vi "Parse Bucket Notification.vi"(11 "Notification Parameters":T1) -> (3 "PUT Data":string)   [LabVIEW 2015, in "NI_AWS_S3.lvlib"]
uses:
  NI_AWS_S3.lvlib
  Notification Configuration.ctl
  Topic Configuration.ctl
  Event.ctl
  Core/HTTP Request/Name Value Pair.ctl
  Cloud Function Configuration.ctl
  Queue Configuration.ctl
  Core/HTTP Request/HTTP Request.lvclass
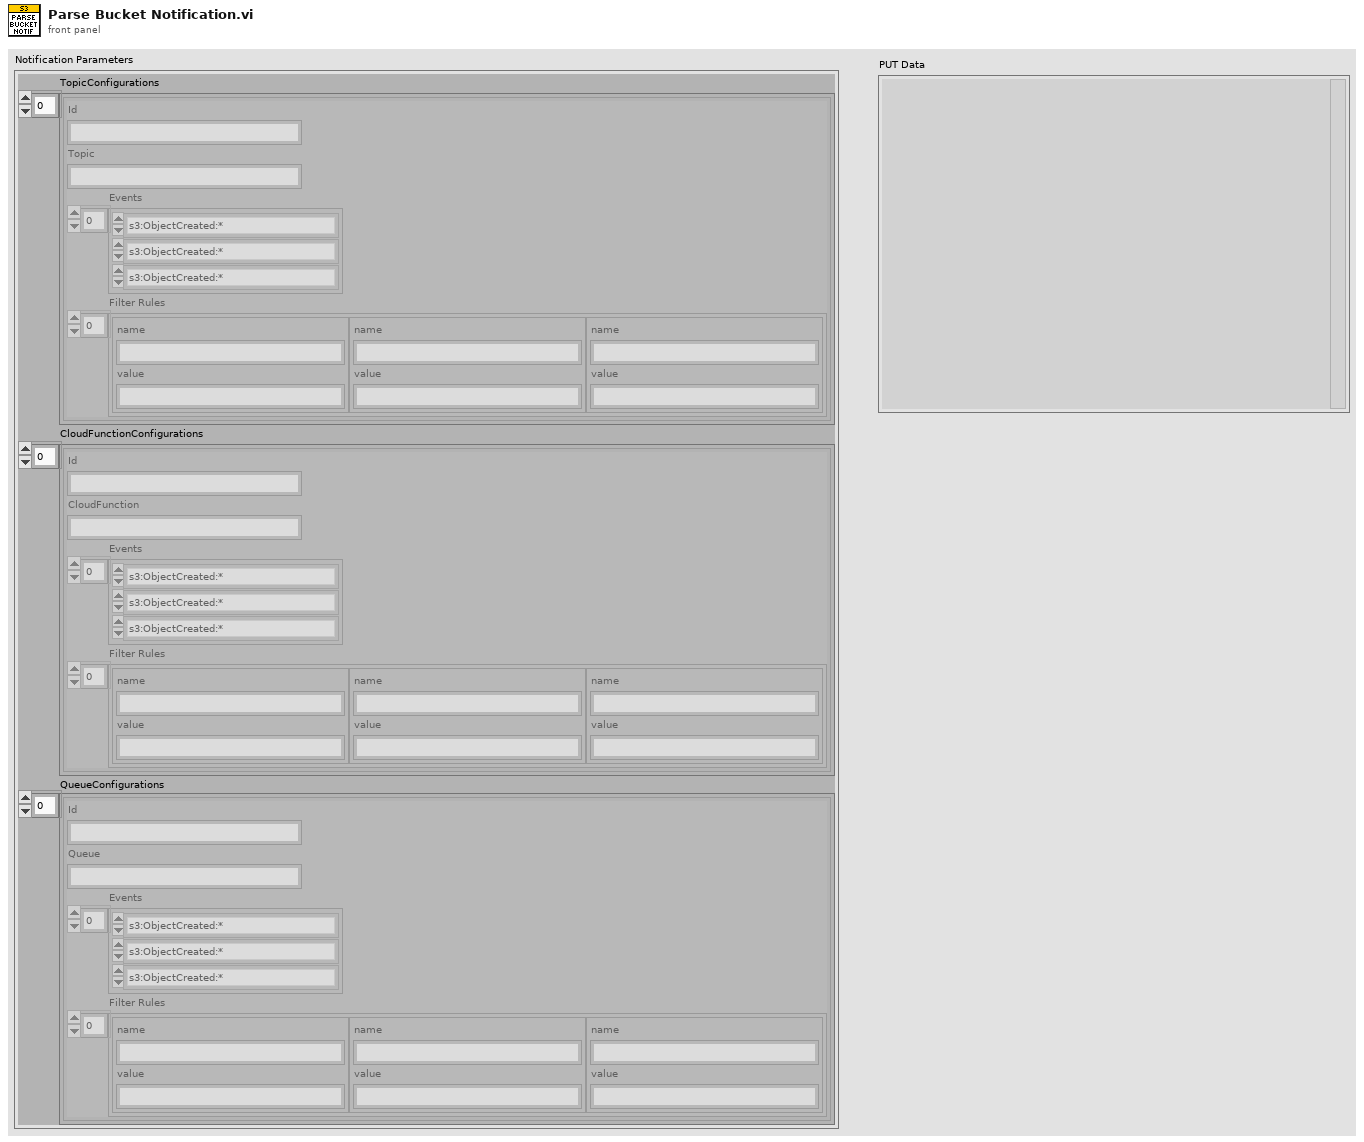
[diagram p1: front panel]
types:
  T1 = typedef "NI_AWS_S3.lvlib/Notification Configuration.ctl" = cluster{"TopicConfigurations":T2[], "CloudFunctionConfigurations":T5[], "QueueConfigurations":T6[]}
  T2 = typedef "NI_AWS_S3.lvlib/Topic Configuration.ctl" = cluster{"Id":string, "Topic":string, "Events":T3[], "Filter Rules":T4[]}
  T3 = typedef "NI_AWS_S3.lvlib/Event.ctl" = enum16{"s3:ObjectCreated:*", "s3:ObjectCreated:Put", "s3:ObjectCreated:Post", "s3:ObjectCreated:Copy", "s3:ObjectCreated:CompleteMultipartUpload", "s3:ObjectRemoved:*", "s3:ObjectRemoved:Delete", "s3:ObjectRemoved:DeleteMarkerCreated", "s3:ReducedRedundancyLostObject"}
  T4 = typedef "NI_AWS_Core.lvlib/HTTP Request.lvclass/Name Value Pair.ctl" = cluster{"name":string, "value":string}
  T5 = typedef "NI_AWS_S3.lvlib/Cloud Function Configuration.ctl" = cluster{"Id":string, "CloudFunction":string, "Events":T3[], "Filter Rules":T4[]}
  T6 = typedef "NI_AWS_S3.lvlib/Queue Configuration.ctl" = cluster{"Id":string, "Queue":string, "Events":T3[], "Filter Rules":T4[]}
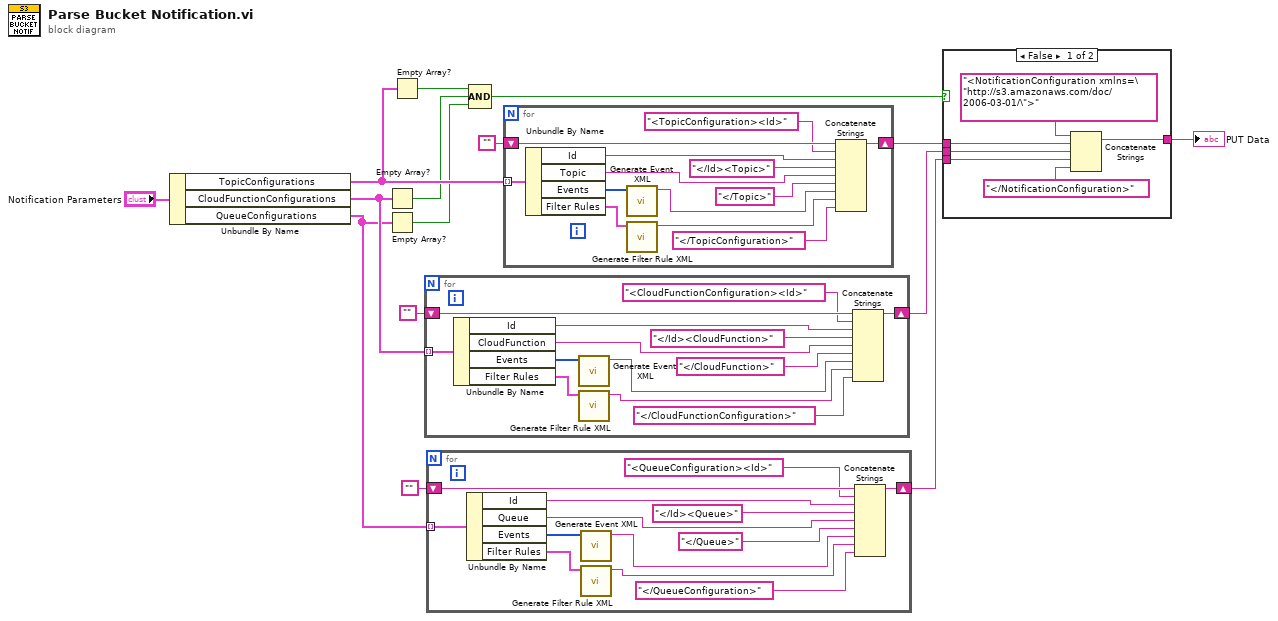
[diagram p0: block diagram]
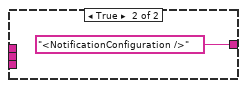
[diagram p2: hidden frame]
diagram:
  n1 = Unbundle By Name("Notification Parameters") -> ("TopicConfigurations"=w12:T2[], "CloudFunctionConfigurations"=w5:T5[], "QueueConfigurations"=w1:T6[])
  n2 = Empty Array?(array=w5) -> (empty?=w10:bool)
  n3 = Empty Array?(array=w1) -> (empty?=w9:bool)
  n4 = Empty Array?(array=w12) -> (empty?=w11:bool)
  n5 = for {
    tunnel: w5 -> [w25] mode=indexing
    shift-right: [w27] -> w4
    shift-left: "" -> [w28]
    n6 = Unbundle By Name(w25) -> ("Id"=w24:string, "CloudFunction"=w22:string, "Events"=w19:T3[], "Filter Rules"=w17:T4[])
    n7 = call "Generate Event XML.vi"("Events"=w19) -> ("Event XML"=w18:string)  [unwired: 10 in]
    n8 = call "Generate Filter Rule XML.vi"("Filter Rules"=w17) -> ("Filter Rule XML"=w16:string)  [unwired: 10 in]
    n9 = Concatenate Strings(w28, "<CloudFunctionConfiguration><Id>", w24, "</Id><CloudFunction>", w22, "</CloudFunction>", w18, w16, "</CloudFunctionConfiguration>") -> (w27:string)
  }
  n10 = for {
    tunnel: w1 -> [w38] mode=indexing
    shift-right: [w40] -> w2
    shift-left: "" -> [w41]
    n11 = Unbundle By Name(w38) -> ("Id"=w37:string, "Queue"=w35:string, "Events"=w32:T3[], "Filter Rules"=w30:T4[])
    n12 = call "Generate Event XML.vi"("Events"=w32) -> ("Event XML"=w31:string)  [unwired: 10 in]
    n13 = call "Generate Filter Rule XML.vi"("Filter Rules"=w30) -> ("Filter Rule XML"=w29:string)  [unwired: 10 in]
    n14 = Concatenate Strings(w41, "<QueueConfiguration><Id>", w37, "</Id><Queue>", w35, "</Queue>", w31, w29, "</QueueConfiguration>") -> (w40:string)
  }
  n15 = Compound Arithmetic op=AND(w11, w10, w9) -> (w8:bool)
  n16 = for {
    tunnel: w12 -> [w51] mode=indexing
    shift-right: [w53] -> w14
    shift-left: "" -> [w54]
    n17 = Unbundle By Name(w51) -> ("Id"=w50:string, "Topic"=w48:string, "Events"=w46:T3[], "Filter Rules"=w44:T4[])
    n18 = call "Generate Event XML.vi"("Events"=w46) -> ("Event XML"=w45:string)  [unwired: 10 in]
    n19 = call "Generate Filter Rule XML.vi"("Filter Rules"=w44) -> ("Filter Rule XML"=w43:string)  [unwired: 10 in]
    n20 = Concatenate Strings(w54, "<TopicConfiguration><Id>", w50, "</Id><Topic>", w48, "</Topic>", w45, w43, "</TopicConfiguration>") -> (w53:string)
  }
  n21 = case shown="False" w8 {
    tunnel: w14 -> [w60 _]
    tunnel: [w59 "<NotificationConfiguration />"] -> w13
    tunnel: w4 -> [w57 _]
    tunnel: w2 -> [w55 _]
    frame False {
      n22 = Concatenate Strings("<NotificationConfiguration xmlns=\"http://s3.amazonaws.com/doc/2006-03-01/\">", w60, w57, w55, "</NotificationConfiguration>") -> (w59:string)
    }
    frame True {
    }
  }
  "PUT Data" <- w13
